vi "AR-AI-read.vi"(7 "number of samples":i32=10, 8 "error in":errorcluster, 11 "AI task in":refnum<k21>) -> (0 "error out":errorcluster, 2 "Data":dbl[](array[numeric]) format="%0.2f", 3 "AI task out":refnum<k21>)   [LabVIEW 2021]
uses:
  <vilib>/DAQmx/read.llb/DAQmx Read (Analog 2D DBL NChan NSamp).vi
  <vilib>/Analysis/baseanly.llb/Mean (DBL).vi
  <vilib>/DAQmx/miscellaneous.llb/DAQmx Fill In Error Info.vi
  <vilib>/Analysis/NI_AALBase.lvlib
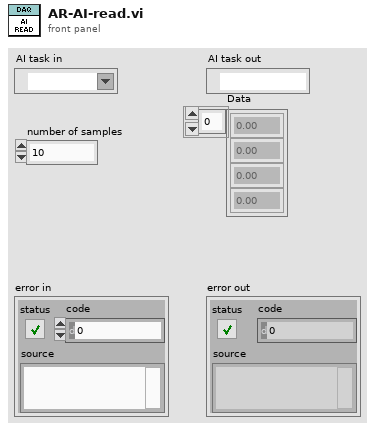
[diagram p1: front panel]
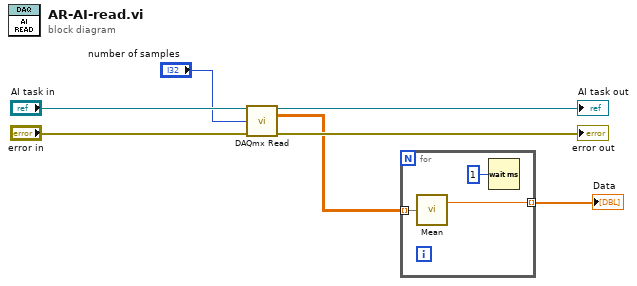
[diagram p0: block diagram]
diagram:
  n1 = call-poly <vilib>:"DAQmx Read.vi"("task/channels in"="AI task in", "number of samples per channel"="number of samples", "error in"="error in") -> ("task out"=→"AI task out":refnum<k21>, "data"=w1:dbl[][], "error out"=→"error out":errorcluster)  [unwired: 10 in]
  n2 = for {
    tunnel: w1 -> [w10] mode=indexing
    tunnel: [w9] -> w2 mode=indexing
    n3 = call-poly <vilib>:"Mean.vi"("X"=w10) -> ("mean"=w9:dbl)  [unwired: 1 out]
    n4 = Wait (ms)(milliseconds to wait=u32 1) -> ()  [unwired: 1 out]
  }
  "Data" <- w2
